vi "To Zero Padded Decimal String.vi"(7 "Required Padding Width":i32, 10 "Number":i32=4) -> (2 "Padded Number":string)   [LabVIEW 2018]
doc: "Takes a <b>Number</b> and produces a zero padded decimal string equal to the width specified by <b>Required Padding Width</b>. (Zeros are padded to the left)."
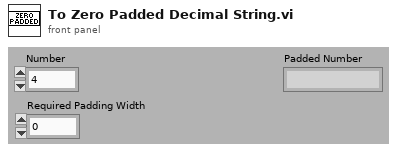
[diagram p1: front panel]
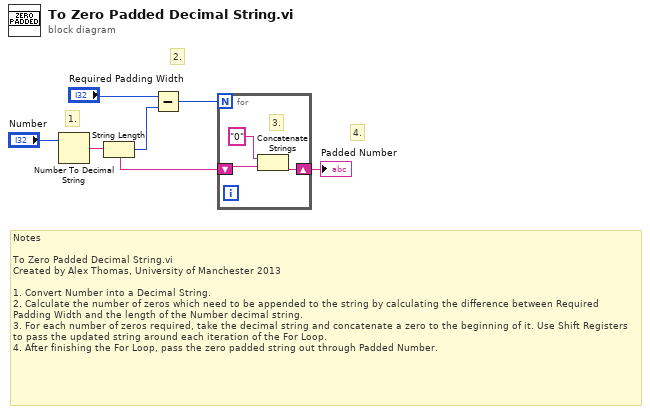
[diagram p0: block diagram]
diagram:
  # "4."
  # "2."
  # "1."
  # "Notes\n\nTo Zero Padded Decimal String.vi\nCreated by Alex Thomas, University of Manchester 2013\n\n1. Convert Number into a Decimal String. \n2. Calculate the number of zeros which need to be appended to the string by calculating the difference between Required Padding Width and the length of the Number decimal string.\n3. For each number of zeros required, take the decimal string and concatenate a zero to the beginning of it. Use Shift Registers to pass the updated string around each iteration of the For Loop.\n4. After finishing the For Loop, pass the zero padded string out through Padded Number."
  n1 = Number To Decimal String(number="Number") -> (decimal integer string=w5:string)  [unwired: 1 in]
  n2 = String Length(string=w5) -> (length=w2:i32)
  n3 = Subtract(x="Required Padding Width", y=w2) -> (x-y=w3:i32)
  n4 = for {
    N: w3 -> [_]
    shift-right: [w7] -> w6
    shift-left: w5 -> [w9]
    # "3."
    n5 = Concatenate Strings("0" ("string"), w9) -> (w7:string)
  }
  "Padded Number" <- w6
